vi "GetState.vi"(8 "error in (no error)":errorcluster, 11 "ControlState in":T1 {"ChainMask" format="0x%02x"}) -> (0 "error out":errorcluster, 2 "State":string, 3 "ControlState out":T1 {"ChainMask" format="0x%02x"})   [LabVIEW 2018, in "ArduinoSerialBling.lvlib"]
uses:
  ArduinoSerialBling.lvlib
  ControlState.ctl
  ConnectionType.ctl
  UdpConnection.ctl
  ChainState.ctl
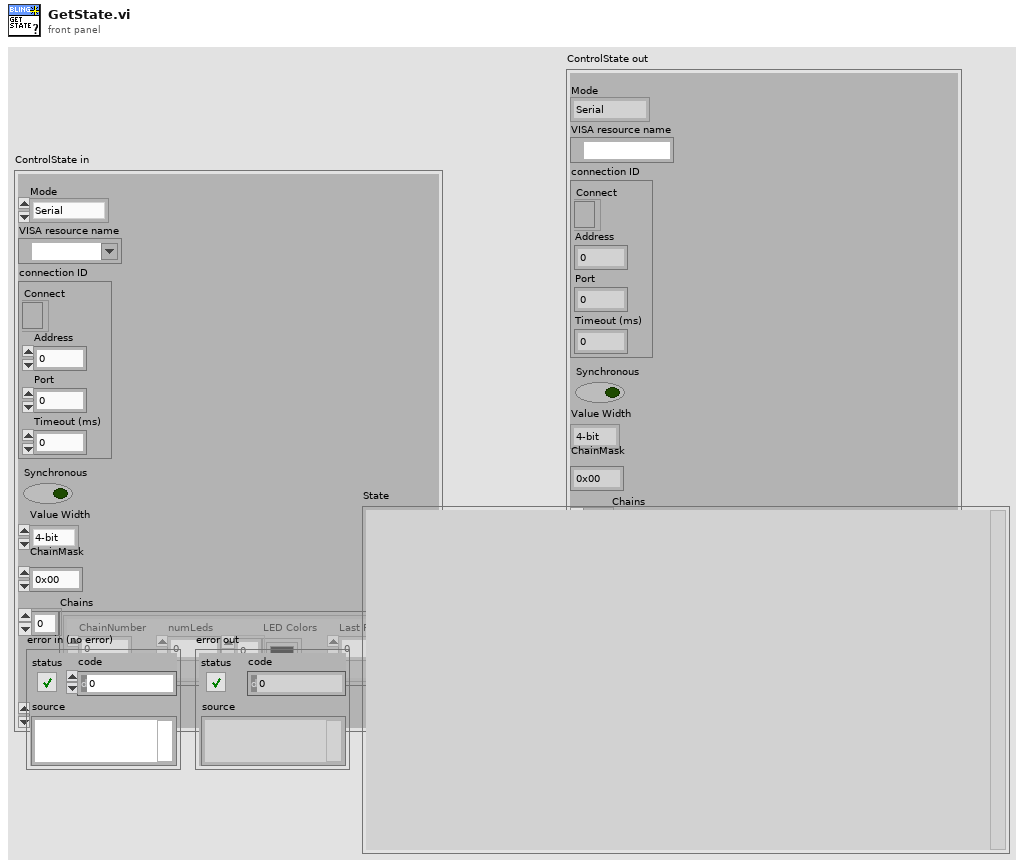
[diagram p1: front panel]
types:
  T1 = typedef "ArduinoSerialBling.lvlib/ControlState.ctl" = cluster{"Mode":T2, "VISA resource name":refnum<visa-resource-name>, "connection ID":T3, "Synchronous":bool, "Value Width":enum16{"4-bit", "8-bit"}, "ChainMask":u8, "Chains":T4[], "Refresh Period (ms)":u32}
  T2 = typedef "ConnectionType.ctl" = enum16{"Serial", "Ethernet", "Offline"}
  T3 = typedef "UdpConnection.ctl" = cluster{"Connect":refnum<k16>, "Address":u32, "Port":u16, "Timeout (ms)":i32}
  T4 = typedef "ArduinoSerialBling.lvlib/ChainState.ctl" = cluster{"ChainNumber":u8, "numLeds":u8, "LED Colors":u32[], "Last Refresh (ms)":u32}
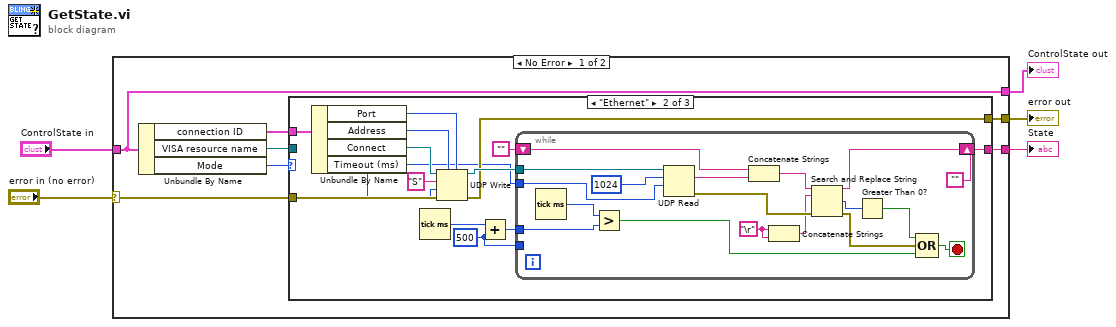
[diagram p0: block diagram]
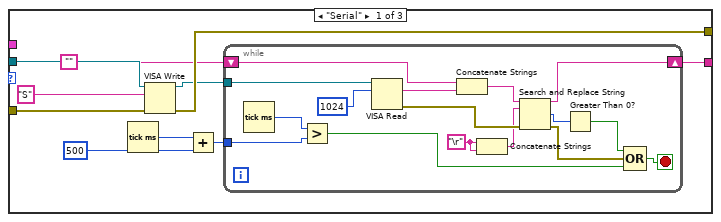
[diagram p2: hidden frame]
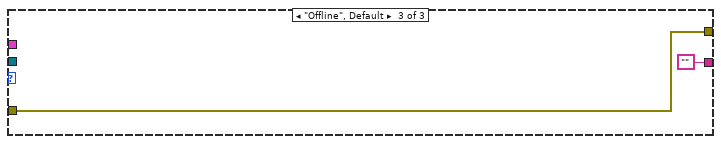
[diagram p3: hidden frame]
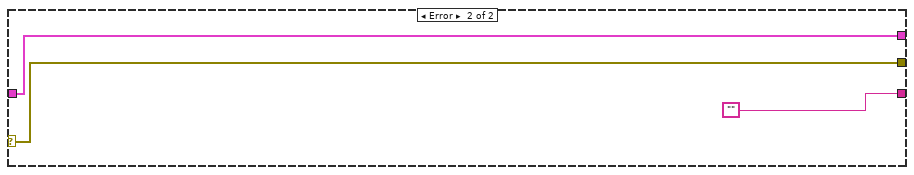
[diagram p4: hidden frame]
diagram:
  n1 = case shown="No Error" "error in (no error)" {
    selector: "error in (no error)" -> [w12 w73]
    tunnel: "ControlState in" -> [w10 w74]
    tunnel: [w8 ""] -> w3
    tunnel: [w9 w73] -> w2
    tunnel: [w10 w74] -> w1
    frame No Error {
      n2 = Unbundle By Name(w10) -> ("connection ID"=w6:T3, "VISA resource name"=w11:refnum<visa-resource-name>, "Mode"=w7:T2)
      n3 = case shown="\"Ethernet\"" w7 {
        tunnel: w12 -> [w22 w46 w71]
        tunnel: w11 -> [w20 _ _]
        tunnel: [w19 w41 w71] -> w9
        tunnel: [w16 "" ""] -> w8
        tunnel: w6 -> [_ w45 _]
        frame "Serial" {
          n4 = Tick Count (ms)() -> (millisecond timer value=w15:u32)
          n5 = VISA Write(VISA resource name=w20, write buffer="S", error in (no error)=w22) -> (VISA resource name out=w18:refnum<visa-resource-name>, error out=w19:errorcluster)  [unwired: 1 out]
          n6 = Add(x=w15, y=u32 500) -> (x+y=w14:u32)
          n7 = while {
            tunnel: w18 -> [w37]
            shift-right: [w32] -> w16
            shift-left: "" -> [w35]
            tunnel: w14 -> [w30]
            stop <- w29 stop-if-true
            w23 = "\r"
            n8 = Tick Count (ms)() -> (millisecond timer value=w31:u32)
            n9 = Greater?(x=w31, y=w30) -> (0:w28:bool)
            n10 = VISA Read(VISA resource name=w37, byte count=u32 1024) -> (read buffer=w36:string, error out=w27:errorcluster)  [unwired: 1 in, 2 out]
            n11 = Concatenate Strings(w35, w36) -> (w33:string)
            n12 = Concatenate Strings(w23, w23) -> (w24:string)
            n13 = Search and Replace String(input string=w33, search string=w24, error in=w27) -> (result string=w32:string, number of replacements=w34:i32, error out=w25:errorcluster)  [unwired: 5 in, 1 out]
            n14 = Greater Than 0?(x=w34) -> (x > 0?=w26:bool)
            n15 = Compound Arithmetic op=OR(w26, w25, w28) -> (w29:bool)
          }
        }
        frame "Ethernet" {
          w40 = u32 500 ("y")
          n16 = Unbundle By Name(w45) -> ("Port"=w43:u16, "Address"=w42:u32, "Connect"=w44:refnum<k16>, "Timeout (ms)"=w39:i32)
          n17 = Tick Count (ms)() -> (millisecond timer value=w48:u32)
          n18 = UDP Write(address=w42, port or service name=w43, connection ID=w44, data in="S" ("write buffer"), 8:w46, 9:w39) -> (error out=w41:errorcluster, 3:w50:refnum<k16>)
          n19 = Add(x=w48, y=w40) -> (x+y=w47:u32)
          n20 = while {
            tunnel: w50 -> [w68]
            shift-right: [w63] -> _
            shift-left: "" -> [w66]
            tunnel: w47 -> [w61]
            tunnel: w40 -> [_]
            tunnel: w39 -> [w53]
            stop <- w60 stop-if-true
            w54 = "\r"
            n21 = Tick Count (ms)() -> (millisecond timer value=w62:u32)
            n22 = Greater?(x=w62, y=w61) -> (0:w59:bool)
            n23 = UDP Read(connection ID=w68, max size (548)=u32 1024 ("byte count"), timeout ms (25000)=w53) -> (data out=w67:string, error out=w58:errorcluster)  [unwired: 1 in, 3 out]
            n24 = Concatenate Strings(w66, w67) -> (w64:string)
            n25 = Concatenate Strings(w54, w54) -> (w55:string)
            n26 = Search and Replace String(input string=w64, search string=w55, error in=w58) -> (result string=w63:string, number of replacements=w65:i32, error out=w56:errorcluster)  [unwired: 5 in, 1 out]
            n27 = Greater Than 0?(x=w65) -> (x > 0?=w57:bool)
            n28 = Compound Arithmetic op=OR(w57, w56, w59) -> (w60:bool)
          }
        }
        frame "Offline", Default {
        }
      }
    }
    frame Error {
    }
  }
  "ControlState out" <- w1
  "error out" <- w2
  "State" <- w3
